vi "WILT Check Current.vi"(10 "L2 Current":dbl, 11 "L1 Current":dbl) -> (1 "L2 Current Out":dbl, 2 "L1 Current Out":dbl, 3 "Agilent Failure":bool)   [LabVIEW 2016]
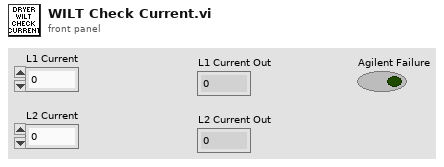
[diagram p1: front panel]
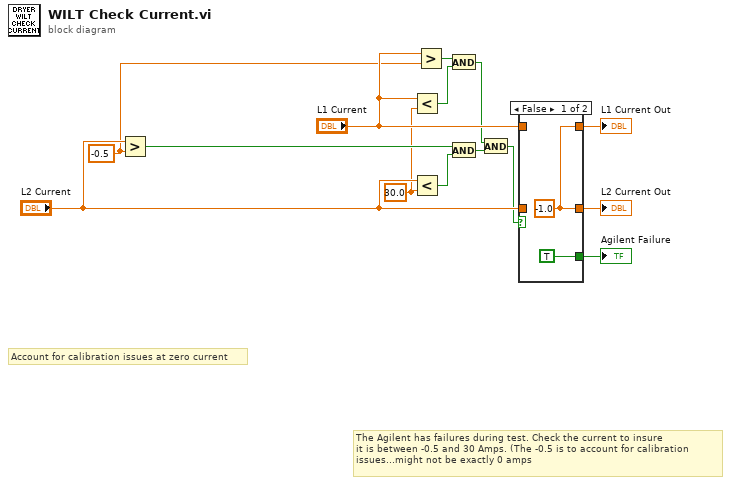
[diagram p0: block diagram]
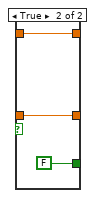
[diagram p2: hidden frame]
diagram:
  w1 = -0.5 ("y")
  w2 = 30.0 ("y")
  # "The Agilent has failures during test. Check the current to insure \nit is between -0.5 and 30 Amps. (The -0.5 is to account for calibration \nissues...might not be exactly 0 amps"
  # "Account for calibration issues at zero current"
  n1 = Greater?(x="L2 Current", y=w1) -> (0:w8:bool)
  n2 = Less?(x="L1 Current", y=w2) -> (x < y?=w10:bool)
  n3 = Less?(x="L2 Current", y=w2) -> (x < y?=w11:bool)
  n4 = Greater?(x="L1 Current", y=w1) -> (0:w6:bool)
  n5 = And(x=w6, y=w10) -> (x .and. y?=w4:bool)
  n6 = And(x=w8, y=w11) -> (x .and. y?=w5:bool)
  n7 = And(x=w4, y=w5) -> (x .and. y?=w3:bool)
  n8 = case shown="False" w3 {
    tunnel: "L1 Current" -> [_ w19]
    tunnel: [w16 w19] -> w12
    tunnel: "L2 Current" -> [_ w18]
    tunnel: [w16 w18] -> w13
    tunnel: [TRUE FALSE] -> w14
    frame False {
      w16 = -1.0
    }
    frame True {
    }
  }
  "Agilent Failure" <- w14
  "L2 Current Out" <- w13
  "L1 Current Out" <- w12
